vi "Latch-Unlatch Button.vi"(0 "Display State In":T1={"Buttons Displayed"=0, "Button States"=[], "Button Size"=0, "Button Style"=enum."Classic", "Active Button"=0, "Force Regen?"=FALSE, "Tip String Ref"=refnum}, 5 "State":bool, 7 "Index":variant, 9 "Container State":T3, 11 "error in (no error)":errorcluster) -> (4 "Display State Out":T1={"Buttons Displayed"=0, "Button States"=[], "Button Size"=0, "Button Style"=enum."Classic", "Active Button"=0, "Force Regen?"=FALSE, "Tip String Ref"=refnum}, 15 "error out":errorcluster)   [LabVIEW 2012, in "Toolbar.xctl"]
doc: "Manually latch or unlatch a specific button as though the user had clicked on it."
uses:
  Toolbar.xctl
  <vilib>/_xctls/Container State.ctl
  Toolbar State.ctl
  Button_Class/Button.lvclass
  Button_Class/Type Defs/Button Style.ctl
  Button_Class/Type Defs/Button Status.ctl
  <vilib>/_xctls/XControlSupport.lvlib
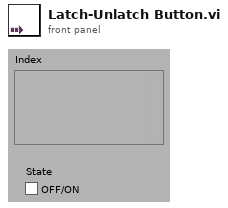
[diagram p1: front panel]
types:
  T1 = typedef "Toolbar.xctl/Toolbar State.ctl" = cluster{"Buttons Displayed":i32, "Button States":refnum<class "Button.lvclass">[], "Button Size":i32, "Button Style":T2, "Active Button":i32, "Force Regen?":bool, "Tip String Ref":refnum<vi>}
  T2 = typedef "Button.lvclass/Button Style.ctl" = enum16{"System", "Modern", "Classic", "Rounded", "Silver", "Ni Theme", "Metallic"}
  T3 = typedef "XControlSupport.lvlib/Container State.ctl" = cluster{"Indicator?":bool, "Run Mode?":bool, " Refnum":refnum<vi>}
  T4 = typedef "Button.lvclass/Button Status.ctl" = enum16{"Off", "Hover", "On", "Disabled"}
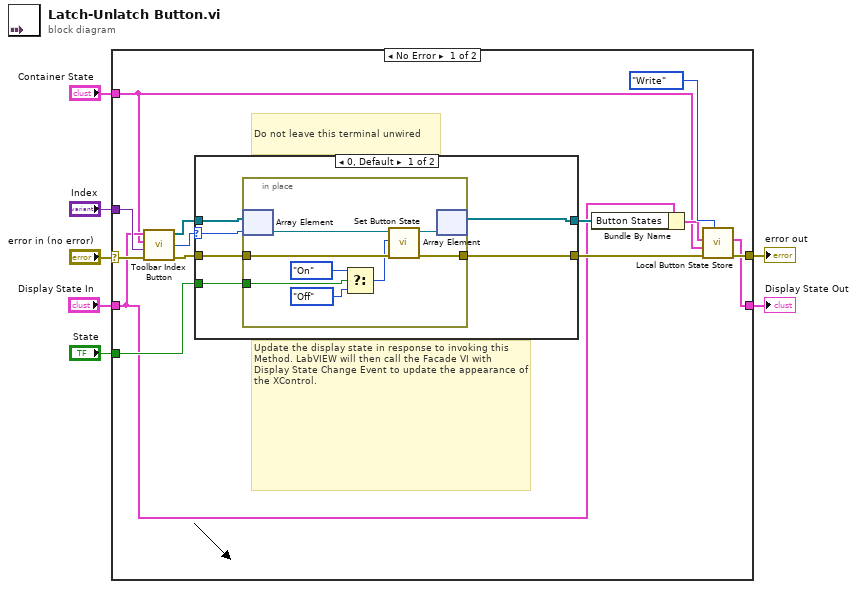
[diagram p0: block diagram]
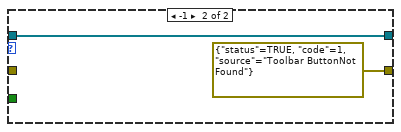
[diagram p2: hidden frame]
diagram:
  n1 = case shown="No Error" "error in (no error)" {
    selector: "error in (no error)" -> [w21 w39]
    tunnel: "Display State In" -> [w9 w38]
    tunnel: [w10 w38] -> w6
    tunnel: "Index" -> [w20 _]
    tunnel: [w14 w39] -> w3
    tunnel: "State" -> [w16 _]
    tunnel: "Container State" -> [w8 _]
    frame No Error {
      # "Do not leave this terminal unwired"
      # "Update the display state in response to invoking this Method. LabVIEW will then call the Facade VI with Display State Change Event to update the appearance of the XControl."
      n2 = call "Toolbar Index Button.vi"("error In (no error)"=w21, "Index"=w20, "Container State"=w8, 10:w9) -> ("error out"=w17:errorcluster, "Output"=w18:refnum<class "Button.lvclass">[], "index of element"=w19:i32)  [unwired: 4 in]
      n3 = case shown="0, Default" w19 {
        selector: w19 -> [w26 _]
        tunnel: [w25 w37] -> w13
        tunnel: w18 -> [w27 w37]
        tunnel: [w23 errorcluster {"status"=TRUE, "code"=1, "source"="Toolbar ButtonNot Found"} ("error out")] -> w15
        tunnel: w17 -> [w24 _]
        tunnel: w16 -> [w22 _]
        frame 0, Default {
          n4 = in-place {
            in-place-border: w24 -> [w33]
            in-place-border: [w32] -> w23
            in-place-border: w22 -> [w31]
            n5 = in-place-array #1(w27, w26) -> (w35:refnum<class "Button.lvclass">)
            n6 = Select(t=Button_Status."On" ("State"), s=w31, f=Button_Status."Off" ("State")) -> (s? t:f=w28:T4)
            n7 = call-dynamic "Set Button State.vi"("error in (no error)"=w33, "State"=w28, "Button in"=w35) -> ("error out"=w32:errorcluster, "Button out"=w34:refnum<class "Button.lvclass">)  [unwired: 7 out]
            n8 = in-place-array #1(w34) -> (w25:refnum<class "Button.lvclass">[])  [unwired: 1 out]
          }
        }
        frame -1 {
        }
      }
      n9 = Bundle By Name(cluster=w9, "Button States"=w13) -> (w11:T1)
      n10 = call "Local Button State Store.vi"("Operation"=enum16{"Read", "Write"}."Write", "error in (no error)"=w15, "Container State"=w8, "Display State In"=w11) -> ("error out"=w14:errorcluster, "Display State Out"=w10:T1)  [unwired: 1 in, 5 out]
    }
    frame Error {
    }
  }
  "Display State Out" <- w6
  "error out" <- w3
